vi "PDCMRAWSave.vi"(0 "DeviceNo":u32, 1 "FileName":string, 2 "Slide Refnum":refnum<vi>, 5 "ChildNo":u32, 11 "error in (no error)":errorcluster, 13 "File_Frame":cluster{"StartFrame":i32, "EndFrame":i32}) -> (15 "error out":errorcluster)   [LabVIEW 2015]
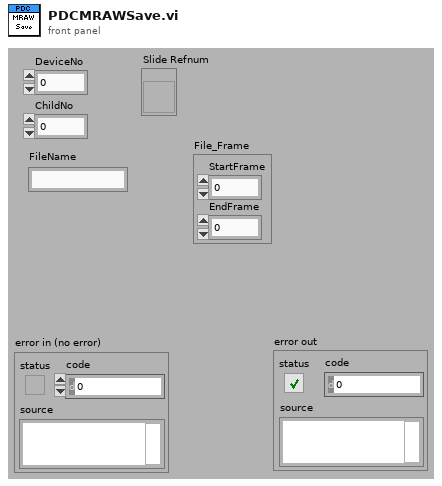
[diagram p1: front panel]
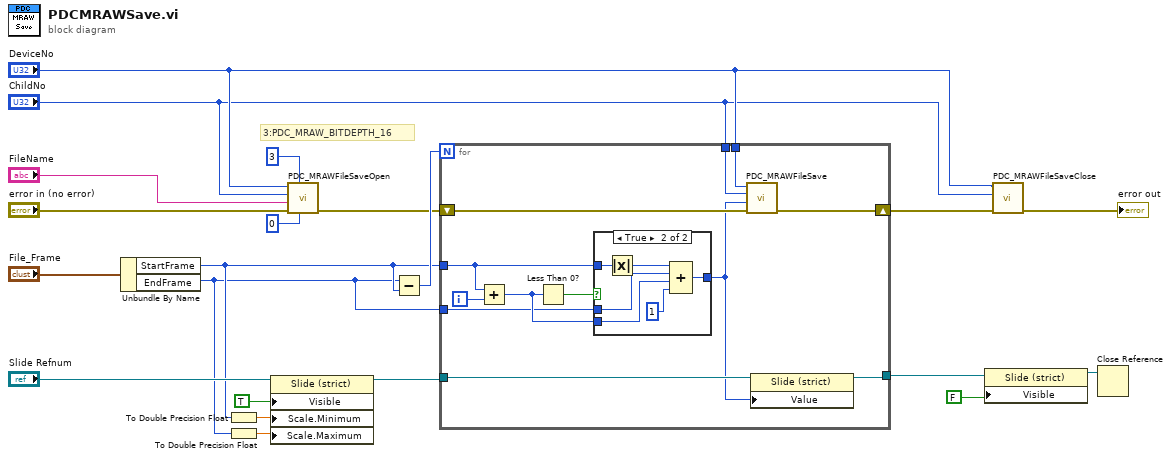
[diagram p0: block diagram]
diagram:
  # "3:PDC_MRAW_BITDEPTH_16"
  n1 = Unbundle By Name("File_Frame") -> ("StartFrame"=w6:i32, "EndFrame"=w5:i32)
  n2 = To Double Precision Float(number=w6) -> (double precision float=w16:dbl)
  n3 = To Double Precision Float(number=w5) -> (double precision float=w17:dbl)
  n4 = property class="Slide (strict)"(reference="Slide Refnum", "Visible"=TRUE ("表示"), "Scale.Minimum"=w16, "Scale.Maximum"=w17) -> (reference out=w12:refnum<vi>)  [unwired: 1 in, 1 out]
  n5 = call "PDC_MRAWFileSaveOpen.vi"("MaxFrameNum"=0, "MRawBitDepth"=u32 3, "error in (no error)"="error in (no error)", "FileName"="FileName", "ChildNo"="ChildNo", "DeviceNo"="DeviceNo") -> ("error out"=w11:errorcluster)  [unwired: 3 in, 2 out]
  n6 = Subtract(x=w5, y=w6) -> (x-y=w14:i32)
  n7 = for {
    N: w14 -> [_]
    tunnel: "DeviceNo" -> [w24]
    tunnel: "ChildNo" -> [w23]
    tunnel: w12 -> [w33]
    tunnel: [w32] -> w18
    shift-right: [w26] -> w4
    shift-left: w11 -> [w25]
    tunnel: w6 -> [w29]
    tunnel: w5 -> [w27]
    i -> [w31]
    n8 = Add(x=w29, y=w31) -> (x+y=w28:i32)
    n9 = Less Than 0?(x=w28) -> (x < 0?=w30:bool)
    n10 = case shown="True" w30 {
      tunnel: w28 -> [w34 w37]
      tunnel: [w34 w35] -> w22
      tunnel: w27 -> [_ w38]
      tunnel: w29 -> [_ w40]
      frame False {
      }
      frame True {
        n11 = Absolute Value(x=w40) -> (abs(x)=w39:i32)
        n12 = Compound Arithmetic op=ADD(w39, w38, w37, 1 ("値")) -> (w35:i32)
      }
    }
    n13 = call "PDC_MRAWFileSave.vi"("error in (no error)"=w25, "FrameNo"=w22, "ChildNo"=w23, "DeviceNo"=w24) -> ("error out"=w26:errorcluster)  [unwired: 5 in, 2 out]
    n14 = property class="Slide (strict)"(reference=w33, "Value"=w22) -> (reference out=w32:refnum<vi>)  [unwired: 1 in, 1 out]
  }
  n15 = property class="Slide (strict)"(reference=w18, "Visible"=FALSE ("表示")) -> (reference out=w20:refnum<vi>)  [unwired: 1 in, 1 out]
  n16 = call "PDC_MRAWFileSaveClose.vi"("error in (no error)"=w4, "ChildNo"="ChildNo", "DeviceNo"="DeviceNo") -> ("error out"=→"error out":errorcluster)  [unwired: 6 in, 2 out]
  n17 = Close Reference(reference=w20) -> ()  [unwired: 1 in, 1 out]
